vi "Labview project.vi"() -> ()   [LabVIEW 2025]
panel:
  in  "Ring 4":u16(ring)
  out "(0 to 19)":dbl
  out "(0 to 19)":dbl
  out "(0 to 19)":dbl
  out "(0 to 19)":dbl
  in  "Ring":u16(ring)
  out "(0 to 19)":dbl
  out "Boolean":bool
  in  "SPIN":bool
  in  "Ring 5":u16(ring)
  in  "Ring 3":u16(ring)
  in  "Ring 2":u16(ring)
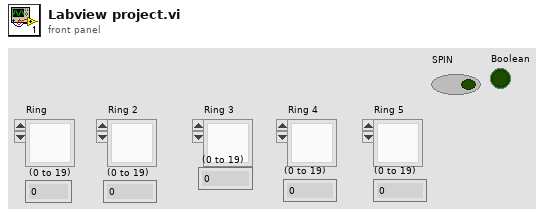
[diagram p1: front panel]
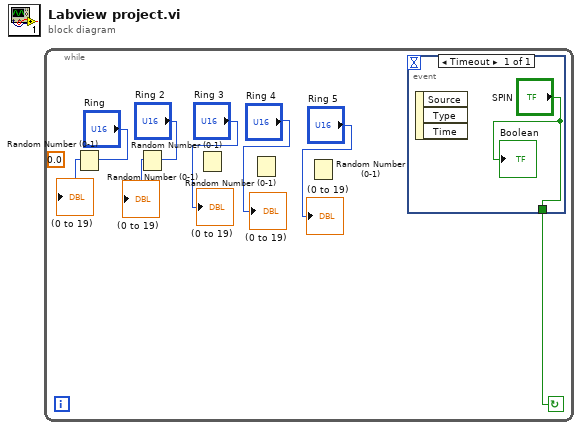
[diagram p0: block diagram]
diagram:
  n1 = while {
    stop <- w6 continue-if-true
    (unwired) 0.0 ("number (0 to 1)")
    n2 = Random Number (0-1) ("Random Number (0,19)")() -> ()  [unwired: 1 out]
    n3 = Random Number (0-1)() -> ()  [unwired: 1 out]
    n4 = Random Number (0-1)() -> ()  [unwired: 1 out]
    n5 = Random Number (0-1)() -> ()  [unwired: 1 out]
    n6 = Random Number (0-1)() -> ()  [unwired: 1 out]
    n7 = event shown="[0] Timeout" {
      selector: _ -> [_]
      dyn-events: _ -> [_]
      timeout: _ -> [_]
      tunnel: ["SPIN"] -> w6
      event Timeout {
        n8 = event-data() -> ()  [unwired: 1 in, 3 out]
        "Boolean" <- "SPIN"
      }
    }
    "(0 to 19)" <- "Ring"
    "(0 to 19)" <- "Ring 2"
    "(0 to 19)" <- "Ring 3"
    "(0 to 19)" <- "Ring 4"
    "(0 to 19)" <- "Ring 5"
  }
